vi "Autonomous Independent.vi"() -> ()   [LabVIEW 2019]
doc: "This VI is called when autonomous begins, and will automatically be terminated when autonomous ends. You can carry out timed or sensor driven robot movement independently without needing to return to the caller."
uses:
  <vilib>/Rock Robotics/WPI/ThirdParty/Phoenix-LabVIEW/Motor Controller/Controls/CTRE_Phoenix_MotorControl_MotionProfileControlMode.ctl
  <vilib>/Rock Robotics/WPI/ThirdParty/Phoenix-LabVIEW/Motor Controller/Controls/CTRE_Phoenix_MotorControl_ControlMode.ctl
  <vilib>/Rock Robotics/WPI/ThirdParty/Phoenix-LabVIEW/Motor Controller/Get/CTRE_Phoenix_MotorController_GetQuadratureData.vi
panel:
  out "Left":i32
  out "Right":i32
  in  "PID":T1={"P"=0.2, "I"=0.0, "D"=0.0, "F"=0.0, "I Zone"=0.0}
  out "Right MP":T2={"Top Buffer Remaining"=0, "Top Buffer Count"=0, "Bottom Buffer Count"=0, "Has Underrun?"=FALSE, "Is Underrun?"=FALSE, "Active Point Valid?"=FALSE, "Is Last?"=FALSE, "Profile Slot Select 0"=0, "Output Enable"=1, "Time Duration (ms)"=50, "Profile Slot Select 1"=0}
  out "Left MP":T2={"Top Buffer Remaining"=0, "Top Buffer Count"=0, "Bottom Buffer Count"=0, "Has Underrun?"=FALSE, "Is Underrun?"=FALSE, "Active Point Valid?"=FALSE, "Is Last?"=FALSE, "Profile Slot Select 0"=0, "Output Enable"=1, "Time Duration (ms)"=0, "Profile Slot Select 1"=0}
  # "0.1"
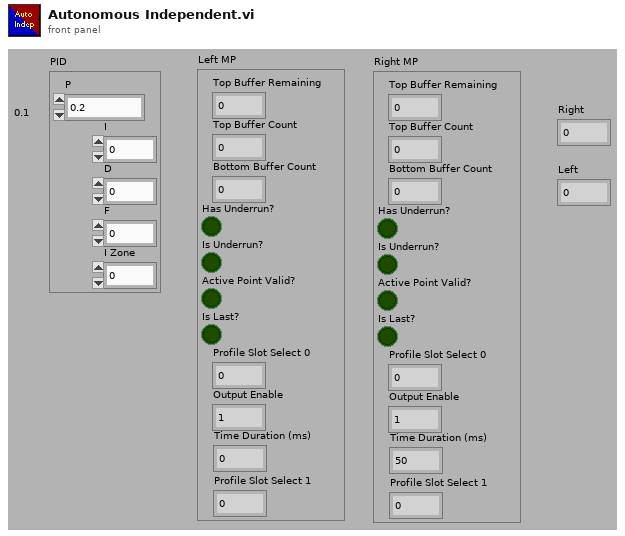
[diagram p1: front panel]
types:
  T1 = cluster{"P":dbl, "I":dbl, "D":dbl, "F":dbl, "I Zone":dbl}
  T2 = cluster{"Top Buffer Remaining":i32, "Top Buffer Count":i32, "Bottom Buffer Count":i32, "Has Underrun?":bool, "Is Underrun?":bool, "Active Point Valid?":bool, "Is Last?":bool, "Profile Slot Select 0":i32, "Output Enable":i32, "Time Duration (ms)":i32, "Profile Slot Select 1":i32}
  T3 = typedef "CTRE_Phoenix_MotorControl_ControlMode.ctl" = u16
  T4 = typedef "CTRE_Phoenix_MotorControl_MotionProfileControlMode.ctl" = u16
  T5 = typedef "WPI_MotorControlDeviceRef.ctl" = cluster{"DeviceStatus":errorcluster, "Type":T6, "PWM":cluster{"PWM Channel":T7, "DeadBand":T8}, "CAN":cluster{"Device Number":u8, "SetOutput VI Ref":variant, "GetOutput VI Ref":variant, "Enable VI Ref":variant, "Disable VI Ref":variant, "Data":variant}, "Invert":bool, "DIO PWM":cluster{"PWM \"Enable\" Channel":T7, "DIOChannel":T9, "PWM Rate":dbl}}
  T6 = typedef "WPI_MotorControlType.ctl" = enum16{"PWM", "CAN", "DIO PWM"}
  T7 = typedef "FPGA_DIOPWMChannel.ctl" = enum8{"PWM 0", "PWM 1", "PWM 2", "PWM 3", "PWM 4", "PWM 5", "PWM 6", "PWM 7", "PWM 8", "PWM 9", "PWM MXP 0", "PWM MXP 1", "PWM MXP 2", "PWM MXP 3", "PWM MXP 4", "PWM MXP 5", "PWM MXP 6", "PWM MXP 7", "PWM MXP 8", "PWM MXP 9", "Invalid"}
  T8 = typedef "WPI_PWMDeadband.ctl" = cluster{"Name":string, "maxPositivePwm":i32, "minPositivePwm":i32, "centerPwm":i32, "maxNegativePwm":i32, "minNegativePwm":i32, "angularRange":u16}
  T9 = typedef "FPGA_DIOChannel.ctl" = enum8{"DIO 0", "DIO 1", "DIO 2", "DIO 3", "DIO 4", "DIO 5", "DIO 6", "DIO 7", "DIO 8", "DIO 9", "DIO MXP 0", "DIO MXP 1", "DIO MXP 2", "DIO MXP 3", "DIO MXP 4", "DIO MXP 5", "DIO MXP 6", "DIO MXP 7", "DIO MXP 8", "DIO MXP 9", "DIO MXP 10", "DIO MXP 11", "DIO MXP 12", "DIO MXP 13", "DIO MXP 14", "DIO MXP 15", "SPI Port CS1", "SPI Port CS2", "SPI Port CS3", "SPI Port MISO", "SPI Port MOSI", "Invalid"}
  T10 = typedef "CTRE_Phoenix_MotorControl_BufferedTrajectoryPointStream_DeviceRef.ctl" = cluster{"Handle":u64, "Library Path":path}
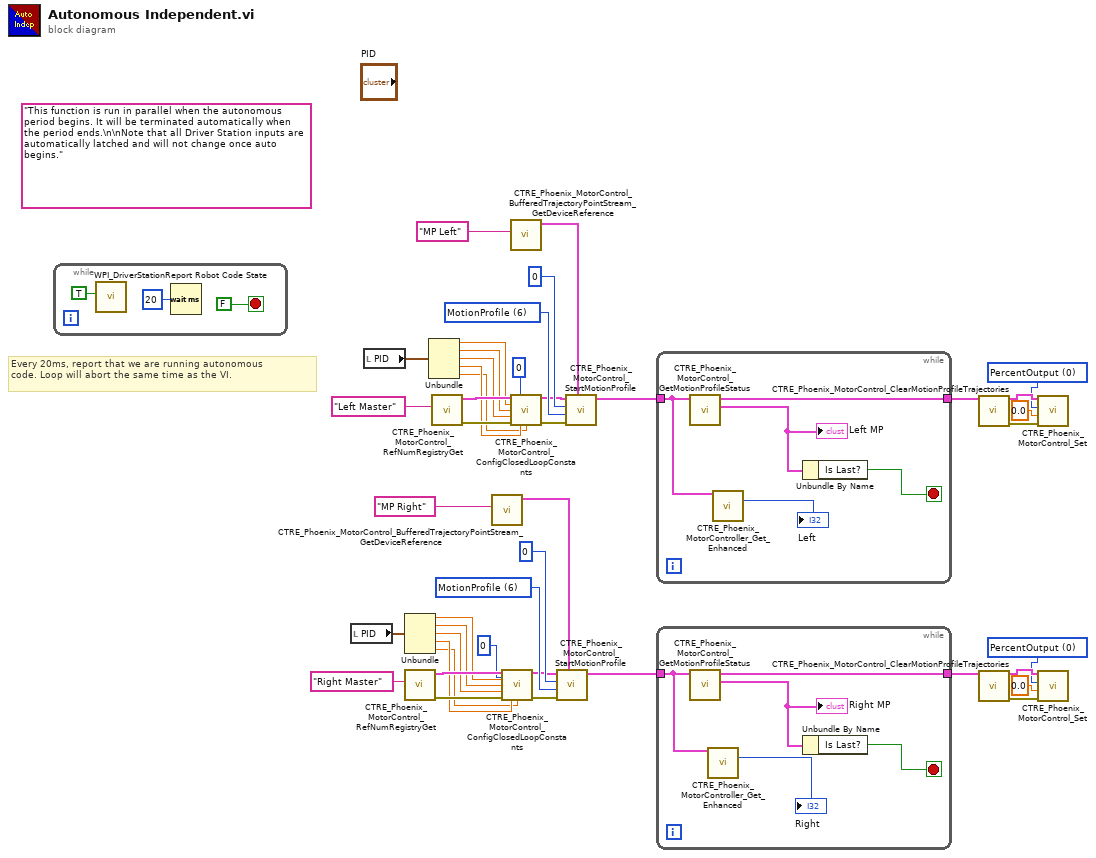
[diagram p0: block diagram]
diagram:
  w25 = T3 0 items=["PercentOutput"=0, "Position"=1, "Velocity"=2, "Current"=3, "Follower"=5, "MotionProfile"=6, "MotionMagic"=7, "MotionProfileArc"=10, "Disabled"=15] ("Control Mode")
  w29 = T3 0 items=["PercentOutput"=0, "Position"=1, "Velocity"=2, "Current"=3, "Follower"=5, "MotionProfile"=6, "MotionMagic"=7, "MotionProfileArc"=10, "Disabled"=15] ("Control Mode")
  w35 = T4 6 items=["MotionProfile"=6, "MotionProfileArc"=10] ("Control Mode")
  w41 = T4 6 items=["MotionProfile"=6, "MotionProfileArc"=10] ("Control Mode")
  (unwired) "This function is run in parallel when the autonomous period begins. It will be terminated automatically when the period ends.\n\nNote that all Driver Station inputs are automatically latched and will not change once auto begins."
  # "Every 20ms, report that we are running autonomous\ncode. Loop will abort the same time as the VI."
  n1 = while {
    stop <- FALSE stop-if-true
    n2 = call <vilib>:"WPI_DriverStationReport Robot Code State.vi"("Autonomous"=TRUE) -> ()  [unwired: 10 in, 1 out]
    n3 = Wait (ms)(milliseconds to wait=u32 20) -> ()  [unwired: 1 out]
  }
  n4 = local read "PID"() -> (w13:T1)
  n5 = local read "PID"() -> (w12:T1)
  n6 = Unbundle(w13) -> ("P"=w18:dbl, "I"=w17:dbl, "D"=w16:dbl, "F"=w15:dbl, "I Zone"=w14:dbl)
  n7 = call <vilib>:"CTRE_Phoenix_MotorControl_RefNumRegistryGet.vi"("refnum name"="Right Master") -> ("error out"=w21:errorcluster, "PhoenixMotorControlDevRef"=w22:T5)  [unwired: 9 in]
  n8 = Unbundle(w12) -> ("P"=w6:dbl, "I"=w5:dbl, "D"=w4:dbl, "F"=w3:dbl, "I Zone"=w2:dbl)
  n9 = call <vilib>:"CTRE_Phoenix_MotorControl_RefNumRegistryGet.vi"("refnum name"="Left Master") -> ("error out"=w7:errorcluster, "PhoenixMotorControlDevRef"=w10:T5)  [unwired: 9 in]
  n10 = call <vilib>:"CTRE_Phoenix_MotorControl_BufferedTrajectoryPointStream_GetDeviceReference.vi"("refnum name"="MP Right") -> ("BufferedTrajectoryPointStream_DevRef"=w38:T10)  [unwired: 9 in, 1 out]
  n11 = call <vilib>:"CTRE_Phoenix_MotorControl_ConfigClosedLoopConstants.vi"("PhoenixMotorControlDevRef"=w22, "slotIdx"=0, "P"=w18, "I"=w17, "D"=w16, "error in (no error)"=w21, "F"=w15, "I Zone"=w14) -> ("PhoenixMotorControlDevRef"=w20:T5, "error out"=w19:errorcluster)  [unwired: 6 in]
  n12 = call <vilib>:"CTRE_Phoenix_MotorControl_BufferedTrajectoryPointStream_GetDeviceReference.vi"("refnum name"="MP Left") -> ("BufferedTrajectoryPointStream_DevRef"=w44:T10)  [unwired: 9 in, 1 out]
  n13 = call <vilib>:"CTRE_Phoenix_MotorControl_ConfigClosedLoopConstants.vi"("PhoenixMotorControlDevRef"=w10, "slotIdx"=0, "P"=w6, "I"=w5, "D"=w4, "error in (no error)"=w7, "F"=w3, "I Zone"=w2) -> ("PhoenixMotorControlDevRef"=w9:T5, "error out"=w8:errorcluster)  [unwired: 6 in]
  n14 = call <vilib>:"CTRE_Phoenix_MotorControl_StartMotionProfile.vi"("BufferedTrajectoryPointStream_DevRef"=w38, "error in"=w19, "Control Mode"=w35, "minBufferedPts"=u32 0, "PhoenixMotorControlDevRef"=w20) -> ("PhoenixMotorControlDevRef"=w33:T5)  [unwired: 5 in, 1 out]
  n15 = call <vilib>:"CTRE_Phoenix_MotorControl_StartMotionProfile.vi"("BufferedTrajectoryPointStream_DevRef"=w44, "error in"=w8, "Control Mode"=w41, "minBufferedPts"=u32 0, "PhoenixMotorControlDevRef"=w9) -> ("PhoenixMotorControlDevRef"=w39:T5)  [unwired: 5 in, 1 out]
  n16 = while {
    tunnel: w39 -> [w49]
    tunnel: [w50] -> w23
    stop <- w51 stop-if-true
    n17 = call <vilib>:"CTRE_Phoenix_MotorControl_GetMotionProfileStatus.vi"("PhoenixMotorControlDevRef"=w49) -> ("Motion Profile Status"=w52:T2, "PhoenixMotorControlDevRef"=w50:T5)  [unwired: 8 in, 1 out]
    "Left MP" <- w52
    n18 = call-poly <vilib>:"CTRE_Phoenix_MotorController_Get_Enhanced.vi"("PhoenixMotorControlDevRef"=w49) -> ("Quadrature Position"=→"Left":i32)  [unwired: 11 in, 3 out]
    n19 = Unbundle By Name(w52) -> ("Is Last?"=w51:bool)
  }
  n20 = while {
    tunnel: w33 -> [w54]
    tunnel: [w55] -> w32
    stop <- w56 stop-if-true
    n21 = call <vilib>:"CTRE_Phoenix_MotorControl_GetMotionProfileStatus.vi"("PhoenixMotorControlDevRef"=w54) -> ("Motion Profile Status"=w57:T2, "PhoenixMotorControlDevRef"=w55:T5)  [unwired: 8 in, 1 out]
    "Right MP" <- w57
    n22 = call-poly <vilib>:"CTRE_Phoenix_MotorController_Get_Enhanced.vi"("PhoenixMotorControlDevRef"=w54) -> ("Quadrature Position"=→"Right":i32)  [unwired: 11 in, 3 out]
    n23 = Unbundle By Name(w57) -> ("Is Last?"=w56:bool)
  }
  n24 = call <vilib>:"CTRE_Phoenix_MotorControl_ClearMotionProfileTrajectories.vi"("PhoenixMotorControlDevRef"=w23) -> ("PhoenixMotorControlDevRef"=w26:T5, "error out"=w27:errorcluster)  [unwired: 13 in]
  n25 = call <vilib>:"CTRE_Phoenix_MotorControl_ClearMotionProfileTrajectories.vi"("PhoenixMotorControlDevRef"=w32) -> ("PhoenixMotorControlDevRef"=w30:T5, "error out"=w31:errorcluster)  [unwired: 13 in]
  n26 = call <vilib>:"CTRE_Phoenix_MotorControl_Set.vi"("error in (no error)"=w27, "Output"=0.0, "Control Mode"=w25, "PhoenixMotorControlDevRef"=w26) -> ()  [unwired: 6 in, 2 out]
  n27 = call <vilib>:"CTRE_Phoenix_MotorControl_Set.vi"("error in (no error)"=w31, "Output"=0.0, "Control Mode"=w29, "PhoenixMotorControlDevRef"=w30) -> ()  [unwired: 6 in, 2 out]
